vi "Dataq REad OLD.vi"(8 "error in (no error)":errorcluster, 10 "reference":refnum<vi>, 11 "VISA Refnum in":refnum<visa-resource-name>) -> (0 "error out":errorcluster, 1 "Outputs":dbl[](array[numeric]), 2 "Waveform Chart":dbl[][](graph)=[[3.57208251953125], [3.55621337890625], [3.55621337890625], [3.55621337890625], [3.56170654296875], [3.56689453125], [3.56170654296875], [3.56170654296875], [3.55621337890625], [3.56170654296875], [3.56170654296875], [3.55621337890625], [3.56689453125], [3.56170654296875], [3.55621337890625], [3.56170654296875], [3.56689453125], [3.56170654296875], [3.56170654296875], [3.56689453125], [3.56170654296875], [3.57208251953125], [3.56170654296875], [3.57208251953125], [3.56170654296875], [3.55621337890625], [3.55621337890625], [3.56689453125], [3.551025390625], [3.56170654296875], [3.55621337890625], [3.56170654296875]], 3 "VISA Refnum out":refnum<visa-resource-name>, 4 "Bytes at Port":u32)   [LabVIEW 2024]
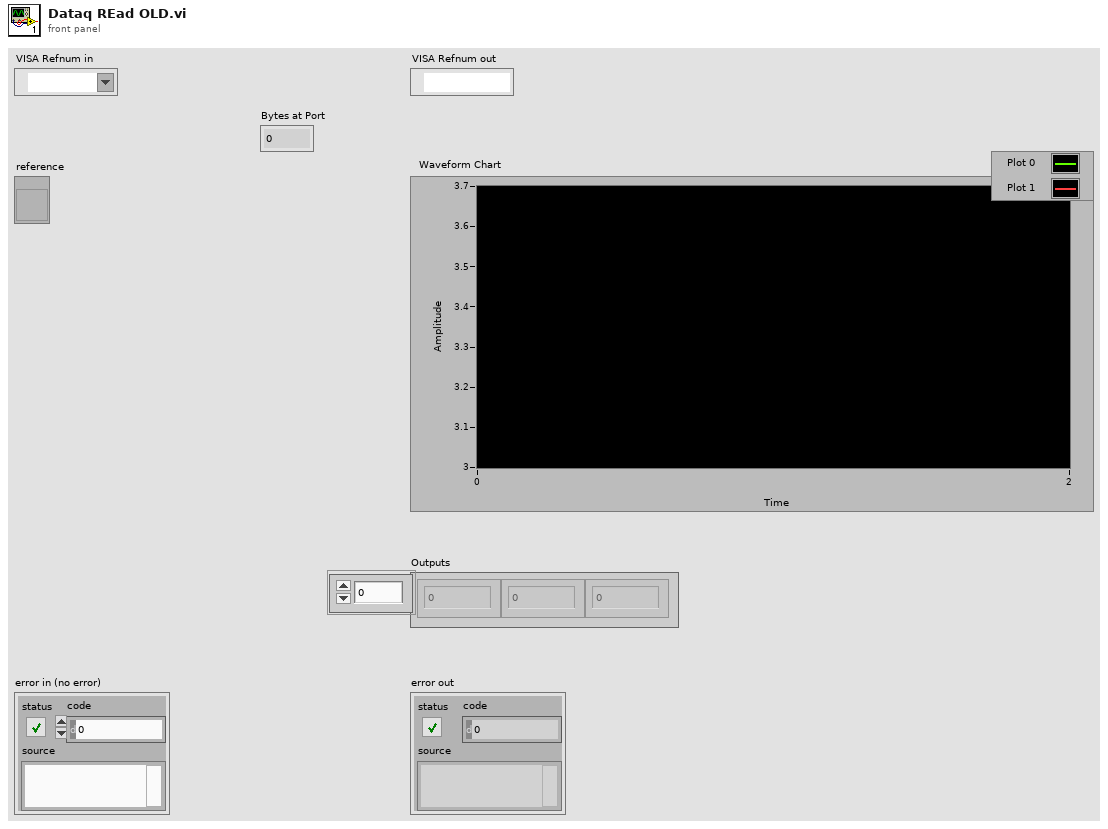
[diagram p1: front panel]
types:
  T1 = enum16{"big-endian, network order", "native, host order", "little-endian"}
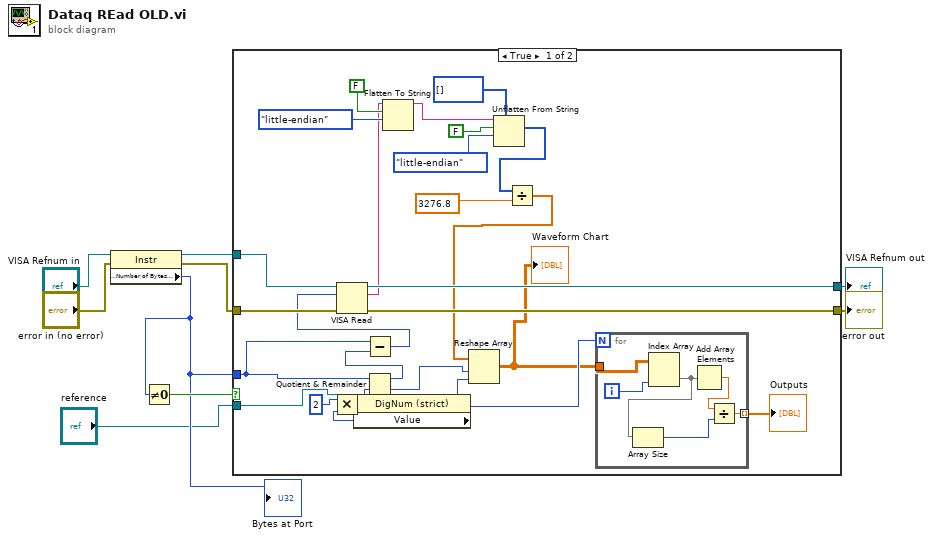
[diagram p0: block diagram]
diagram:
  n1 = property class="Instr"(reference="VISA Refnum in", error in="error in (no error)") -> (reference out=w5:refnum<visa-resource-name>, error out=w7:errorcluster, "Serial Settings:Number of Bytes at Serial Port"=w8:u32)
  "Bytes at Port" <- w8
  n2 = Not Equal To 0?(x=w8) -> (x != 0?=w9:bool)
  n3 = case shown="True" w9 {
    tunnel: [w32 w40] -> w2
    tunnel: w7 -> [w33 w41]
    tunnel: [w28 w41] -> w3
    tunnel: w5 -> [w13 w40]
    tunnel: w8 -> [w12 _]
    tunnel: "reference" -> [w10 _]
    frame True {
      n4 = property class="DigNum (strict)"(reference=w10) -> ("Value"=w15:i32)  [unwired: 1 in, 2 out]
      n5 = Multiply(x=2, y=w15) -> (x*y=w16:i32)
      n6 = Quotient & Remainder(x=w12, y=w16) -> (x-y*floor(x/y)=w30:u32, floor(x/y)=w18:u32)
      n7 = Subtract(x=w12, y=w30) -> (x-y=w29:u32)
      n8 = VISA Read(VISA resource name=w13, byte count=w29, error in (no error)=w33) -> (VISA resource name out=w32:refnum<visa-resource-name>, read buffer=w22:string, error out=w28:errorcluster)  [unwired: 1 out]
      n9 = Flatten To String(anything=w22, prepend array or string size? (T)=FALSE, byte order (0:big-endian, network order)=T1."little-endian") -> (data string=w23:string)  [unwired: 1 in, 2 out]
      n10 = Unflatten From String(type=i16[] [], binary string=w23, data includes array or string size? (T)=FALSE, byte order (0:big-endian, network order)=T1."little-endian") -> (value=w21:i16[])  [unwired: 1 in, 2 out]
      n11 = Divide(x=w21, y=3276.8) -> (x/y=w19:dbl[])
      n12 = Reshape Array(w19, w18, w15) -> (w14:dbl[][])
      "Waveform Chart" <- w14
      n13 = for {
        N: w15 -> [_]
        tunnel: w14 -> [w39]
        tunnel: [w36] -> w11 mode=indexing
        i -> [w34]
        n14 = Index Array(array=w39, index (col)=w34) -> (element=w35:dbl[])  [unwired: 1 in]
        n15 = Array Size(array=w35) -> (size(s)=w37:i32)
        n16 = Add Array Elements(numeric array=w35) -> (sum=w38:dbl)
        n17 = Divide(x=w38, y=w37) -> (x/y=w36:dbl)
      }
      "Outputs" <- w11
    }
    frame False {
    }
  }
  "error out" <- w3
  "VISA Refnum out" <- w2
